vi "power.vi"(8 "error in (no error)":errorcluster, 11 "BasicRemote in":refnum<class "BasicRemote.lvclass">) -> (0 "error out":errorcluster, 3 "BasicRemote out":refnum<class "BasicRemote.lvclass">)   [LabVIEW 2017, in "BasicRemote.lvclass"]
uses:
  BasicRemote.lvclass
  BasicRemote.lvclass/BasicRemote.ctl
  Device Class/Device.lvclass
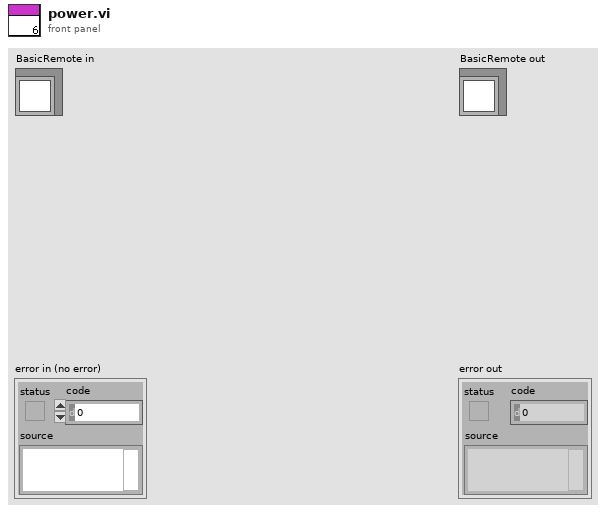
[diagram p1: front panel]
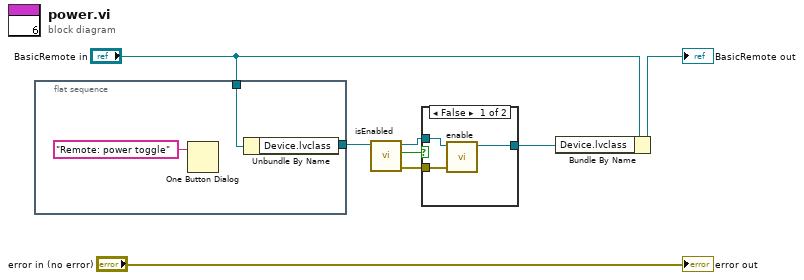
[diagram p0: block diagram]
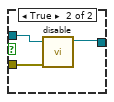
[diagram p2: hidden frame]
diagram:
  n1 = flat-sequence {
    tunnel: "BasicRemote in" -> [w10]
    tunnel: [w9] -> w6
    frame #0 {
      n2 = One Button Dialog(message="Remote: power toggle") -> ()  [unwired: 1 in, 1 out]
      n3 = Unbundle By Name(w10) -> ("Device.lvclass"=w9:refnum<class "Device.lvclass">)
    }
  }
  n4 = call-dynamic "isEnabled.vi"("Device in"=w6) -> ("error out"=w3:errorcluster, "on"=w5:bool, "Device out"=w4:refnum<class "Device.lvclass">)  [unwired: 8 in]
  n5 = case shown="False" w5 {
    tunnel: w4 -> [w14 w17]
    tunnel: w3 -> [w13 w16]
    tunnel: [w12 w15] -> w1
    frame False {
      n6 = call-dynamic "enable.vi"("error in (no error)"=w13, "Device in"=w14) -> ("Device out"=w12:refnum<class "Device.lvclass">)  [unwired: 8 in, 1 out]
    }
    frame True {
      n7 = call-dynamic "disable.vi"("error in (no error)"=w16, "Device in"=w17) -> ("Device out"=w15:refnum<class "Device.lvclass">)  [unwired: 8 in, 1 out]
    }
  }
  n8 = Bundle By Name(cluster="BasicRemote in", "Device.lvclass"=w1) -> (→"BasicRemote out":refnum<class "BasicRemote.lvclass">)
  "error out" <- "error in (no error)"
